vi "TypeConv_Obtain Writer.vi"(10 "Class Name":string, 11 "Writer Map":variant) -> (2 "Abstract Param Writer out":refnum<class "Abstract Param Writer.lvclass">, 3 "Writer Map Dup":variant)   [LabVIEW 2013]
doc: "Copyright (c) 2016 Sze Howe Koh\n\nThis Source Code Form is subject to the terms of the Mozilla Public License, v. 2.0. If a copy of the MPL was not distributed with this file, You can obtain one at http://mozilla.org/MPL/2.0/."
uses:
  Abstract Param Writer/Abstract Param Writer.lvclass
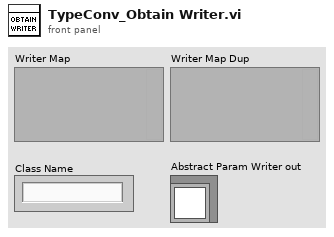
[diagram p1: front panel]
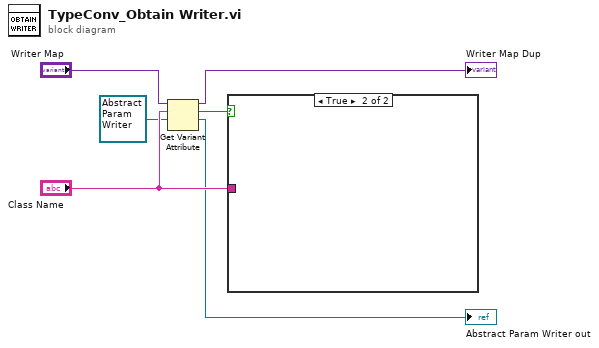
[diagram p0: block diagram]
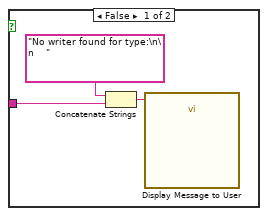
[diagram p2: hidden frame]
diagram:
  n1 = Get Variant Attribute(Variant="Writer Map", name="Class Name", default value (empty Variant)=refnum<class "Abstract Param Writer.lvclass"> refnum ("Abstract Param Writer.lvclass")) -> (duplicate Variant=→"Writer Map Dup":variant, found=w5:bool, value=→"Abstract Param Writer out":refnum<class "Abstract Param Writer.lvclass">)  [unwired: 1 in, 1 out]
  n2 = case shown="True" w5 {
    tunnel: "Class Name" -> [w8 _]
    frame False {
      n3 = Concatenate Strings("No writer found for type:\n\n    ", w8) -> (w7:string)
      n4 = call "Display Message to User"("Message"=w7) -> ()  [unwired: 9 in, 2 out]
    }
    frame True {
    }
  }
